vi "Check For Read Only Error.vi"(8 "error in (no error)":errorcluster, 10 "Write?":bool, 11 "Abs_Value in":refnum<class "Abs_Value.lvclass">) -> (0 "error out":errorcluster, 3 "Abs_Value out":refnum<class "Abs_Value.lvclass">)   [LabVIEW 2021, in "Omni_Bus.lvclass"]
uses:
  Omni_Bus.lvclass
  <vilib>/TSA/Abstract Data Classes/Abs_Types/Value/Abs_Value.lvclass
  <vilib>/Utility/error.llb/Error Cluster From Error Code.vi
  <vilib>/ErrorRing/Error Ring.xnode
  Omni_Bus.lvclass/Omni_Bus.ctl
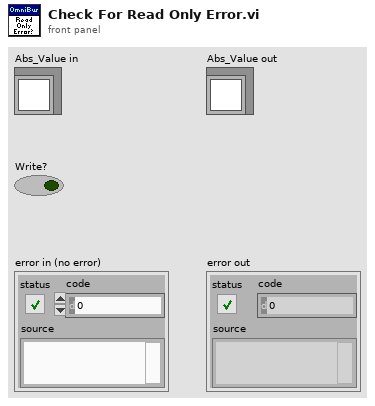
[diagram p1: front panel]
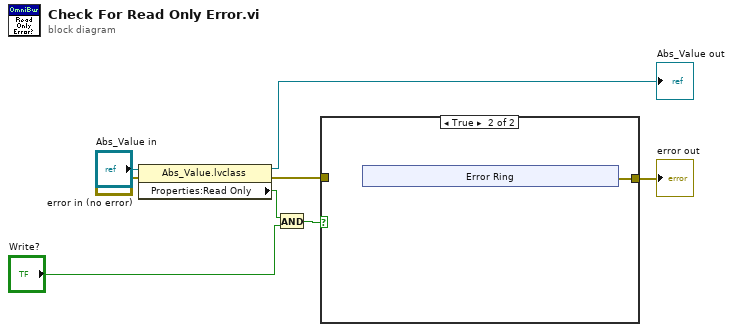
[diagram p0: block diagram]
diagram:
  n1 = property class="Abs_Value.lvclass"(reference="Abs_Value in", error in="error in (no error)") -> (reference out=→"Abs_Value out":refnum<class "Abs_Value.lvclass">, error out=w7:errorcluster, "Properties:Read Only"=w4:bool)
  n2 = And(x=w4, y="Write?") -> (x .and. y?=w6:bool)
  n3 = case shown="True" w6 {
    tunnel: w7 -> [w9 _]
    tunnel: [w9 w10] -> w8
    frame False {
    }
    frame True {
      n4 = xnode "Error Ring"() -> ("error out"=w10:errorcluster)
    }
  }
  "error out" <- w8
